vi "Read Test Executive Ref.vi"(11 "Test Executive in":refnum<class "Test Executive.lvclass">) -> (2 "Test Executive Ref":refnum<data-value>, 3 "Test Executive out":refnum<class "Test Executive.lvclass">)   [LabVIEW 2020, in "Test Executive.lvlib" / "Test Executive.lvclass"]
uses:
  <vilib>/gpm_packages/@cs/test-executive/Source/Test Executive/TestExecutive/Test Executive.lvclass
  <vilib>/gpm_packages/@cs/linked-list/Source/Linked List/ILinkedList/ILinked List.lvclass
  <vilib>/gpm_packages/@cs/test-executive/Source/Test Executive/TestExecutive/Test Executive.lvclass/Test Executive.ctl
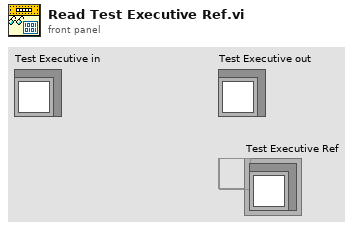
[diagram p1: front panel]
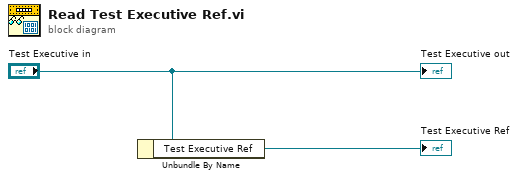
[diagram p0: block diagram]
diagram:
  n1 = Unbundle By Name("Test Executive in") -> ("Test Executive Ref"=→"Test Executive Ref":refnum<data-value>)
  "Test Executive out" <- "Test Executive in"
